vi "XiXi-1(Add U8).vi"(10 "X[-1]":u8, 11 "Xi":u8[](array[numeric])) -> (3 "Yi":u8[](array[numeric]))   [LabVIEW 2012]
doc: "Calculate sums of consecutive array elements. 0th element of output is equal to x(0)+ x(-1), where x(-1) is an optional scalar input that defaults to zero."
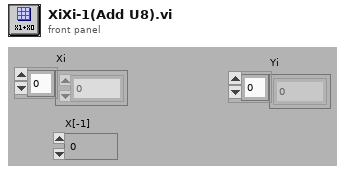
[diagram p1: front panel]
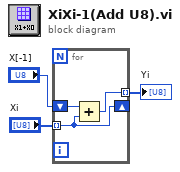
[diagram p0: block diagram]
diagram:
  n1 = for {
    shift-right: [w5] -> _
    shift-left: "X[-1]" -> [w6]
    tunnel: "Xi" -> [w5] mode=indexing
    tunnel: [w4] -> w1 mode=indexing
    n2 = Add(x=w6, y=w5) -> (x+y=w4:u8)
  }
  "Yi" <- w1
